vi "add channel to configuration.vi"(8 "error in":errorcluster, 10 "TBM channel in":refnum<class "TBM channel.lvclass">, 11 "Shared Library Module configuration in":refnum<class "Shared Library Module configuration.lvclass">) -> (0 "error out":errorcluster, 3 "Shared Library Module configuration out":refnum<class "Shared Library Module configuration.lvclass">)   [LabVIEW 2013, in "Shared Library Module configuration.lvclass"]
doc: "Platypus Framework 1.0.1.60\nNI Systems Engineering - National Instruments"
uses:
  Shared Library Module configuration.lvclass
  <vilib>/NI/Tag Bus Module Framework/channel/TBM channel.lvclass
  <vilib>/NI/Tag Bus/tag/tag descriptor.lvclass/tag descriptor.ctl
  Shared Library Module configuration.lvclass/Shared Library Module configuration.ctl
  <vilib>/NI/Tag Bus/tag/tag descriptor.lvclass
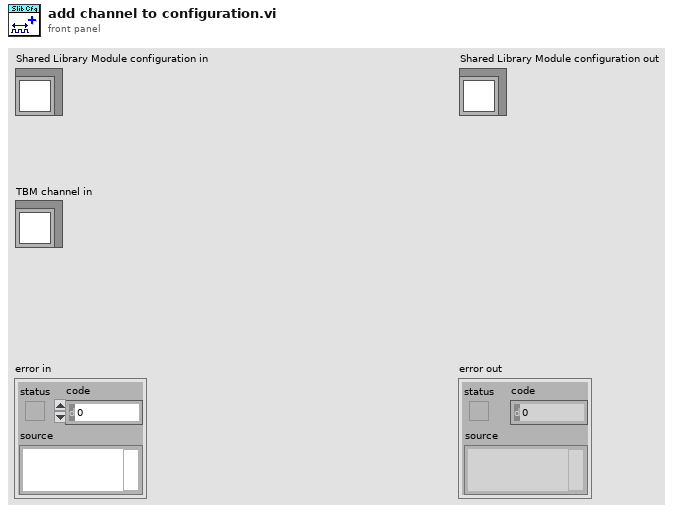
[diagram p1: front panel]
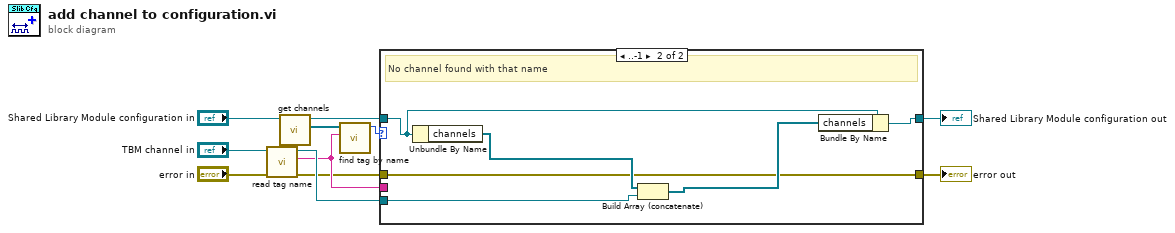
[diagram p0: block diagram]
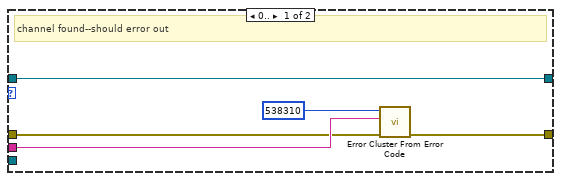
[diagram p2: hidden frame]
diagram:
  n1 = call <vilib>:"read tag name.vi"("error in"="error in", "system tag in"="TBM channel in") -> ("error out"=w2:errorcluster, "name"=w3:string, "system tag out"=w10:refnum<class "TBM channel.lvclass">)  [unwired: 7 in]
  n2 = call-dynamic "get channels.vi"("Shared Library Module configuration in"="Shared Library Module configuration in") -> ("channels"=w5:refnum<class "TBM channel.lvclass">[], "Shared Library Module configuration out"=w11:refnum<class "Shared Library Module configuration.lvclass">)  [unwired: 9 in]
  n3 = call <vilib>:"find tag by name.vi"("name"=w3, "tags in"=w5) -> ("index"=w4:i32)  [unwired: 9 in]
  n4 = case shown="..-1" w4 {
    tunnel: [w16 w17] -> w8
    tunnel: w3 -> [w14 _]
    tunnel: w2 -> [w13 w17]
    tunnel: w11 -> [w12 w21]
    tunnel: w10 -> [_ w22]
    tunnel: [w12 w20] -> w7
    frame 0.. {
      # "channel found--should error out"
      n5 = call <vilib>:"Error Cluster From Error Code.vi"("error in (no error)"=w13, "error message (\"\")"=w14, "error code (0)"=538310) -> ("error out"=w16:errorcluster)  [unwired: 6 in]
    }
    frame ..-1 {
      # "No channel found with that name"
      n6 = Unbundle By Name(w21) -> ("channels"=w19:refnum<class "TBM channel.lvclass">[])
      n7 = Build Array (concatenate)(w19, w22) -> (w18:refnum<class "TBM channel.lvclass">[])
      n8 = Bundle By Name(cluster=w21, "channels"=w18) -> (w20:refnum<class "Shared Library Module configuration.lvclass">)
    }
  }
  "error out" <- w8
  "Shared Library Module configuration out" <- w7
